vi "merge hydrolysis files.vi"(7 "current_starttime":i32, 8 "error in (no error)":errorcluster, 9 "filename":string, 10 "reactor_names":string, 11 "dir":string) -> (0 "error out":errorcluster, 3 "function return":string)   [LabVIEW 2019, in "libFileFunctions.lvlib"]
doc: "const char* merge_hydrolysis_files(const char* dir, const char* reactor_names, const char* filename, int current_starttime);"
uses:
  libFileFunctions.lvlib
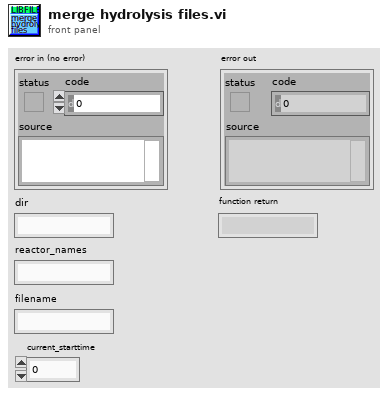
[diagram p1: front panel]
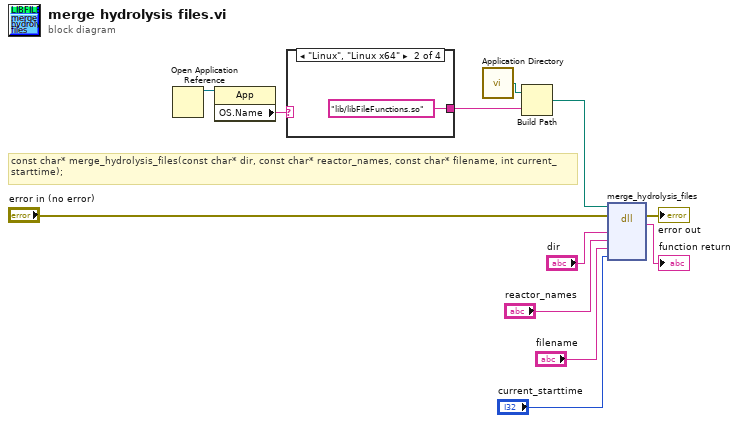
[diagram p0: block diagram]
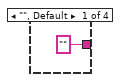
[diagram p2: hidden frame]
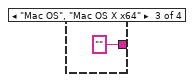
[diagram p3: hidden frame]
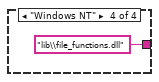
[diagram p4: hidden frame]
diagram:
  # "const char* merge_hydrolysis_files(const char* dir, const char* reactor_names, const char* filename, int current_starttime);"
  n1 = Open Application Reference() -> (3:w5:refnum<vi>)  [unwired: 4 in, 1 out]
  n2 = property class="App"(reference=w5) -> ("OS.Name"=w4:string)  [unwired: 1 in, 2 out]
  n3 = case shown="\"Linux\", \"Linux x64\"" w4 {
    tunnel: ["" ("return type") "lib/libFileFunctions.so" ("name or relative path") "" ("return type") "lib\\file_functions.dll" ("name or relative path")] -> w3
    frame "", Default {
    }
    frame "Linux", "Linux x64" {
    }
    frame "Mac OS", "Mac OS X x64" {
    }
    frame "Windows NT" {
    }
  }
  n4 = call <vilib>:"Application Directory.vi"() -> ("Application Directory"=w2:path)
  n5 = Build Path(base path=w2, name or relative path=w3) -> (appended path=w1:path)
  n6 = dll-call lib="home/paul/Schreibtisch/Biogas_plant_setup/LabView/lib/libFileFunctions/libFileFunctions.*" fn="merge_hydrolysis_files"(path in=w1, error in="error in (no error)", "dir"="dir", "reactor_names"="reactor_names", "filename"="filename", "current_starttime"="current_starttime") -> (error out=→"error out":errorcluster, "return type"=→"function return":string)  [unwired: 5 in, 1 out]
